vi "gu_message_box.vi"(7 "Title":T3, 8 "error in":errorcluster, 9 "Icon":T1, 10 "Choice":T2, 11 "Message":T3) -> (0 "error out":errorcluster, 3 "Button":T4=enum."Cancel")   [LabVIEW 2020, in "G-Unicode.lvlib"]
uses:
  G-Unicode.lvlib
  Dialog & User Interface/Message Box/Message Box Dialog Button.ctl
  Types/Encoded UTF-8 String.ctl
  Dialog & User Interface/Message Box/Message Box Dialog Type.ctl
  Dialog & User Interface/Message Box/Message Box Icon Type.ctl
  <vilib>/Utility/file.llb/Application Directory.vi
  <vilib>/Utility/error.llb/Error Cluster From Error Code.vi
  lib/g_unicode_32.dll
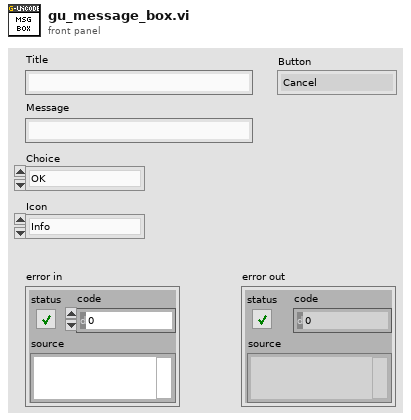
[diagram p1: front panel]
types:
  T1 = typedef "G-Unicode.lvlib/Message Box Icon Type.ctl" = enum16{"Info", "Warning", "Error", "Question"}
  T2 = typedef "G-Unicode.lvlib/Message Box Dialog Type.ctl" = enum32{"OK", "OK/Cancel", "Yes/No", "Yes/No/Cancel", "Retry/Cancel", "Abort/Retry/Ignore"}
  T3 = typedef "G-Unicode.lvlib/Encoded UTF-8 String.ctl" = string
  T4 = typedef "G-Unicode.lvlib/Message Box Dialog Button.ctl" = enum32{"OK", "Yes", "No", "Abort", "Retry", "Ignore", "Cancel"}
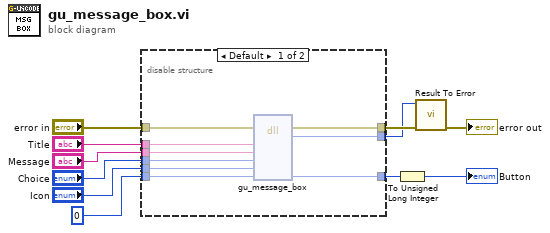
[diagram p0: block diagram]
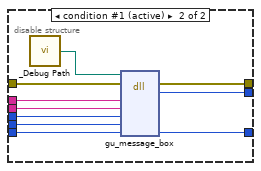
[diagram p2: hidden frame]
diagram:
  n1 = disable-structure shown="Default" {
    disable-tunnel: [w20 w30] -> w11
    disable-tunnel: [w14 w22] -> w10
    disable-tunnel: "Title" -> [w19 w29]
    disable-tunnel: "error in" -> [w18 w28]
    disable-tunnel: "Message" -> [w17 w27]
    disable-tunnel: "Choice" -> [w16 w26]
    disable-tunnel: "Icon" -> [w15 w25]
    disable-tunnel: [w13 w21] -> w2
    disable-tunnel: 0 ("user_selection") -> [w12 w23]
    frame condition #0 {
      n2 = dll-call lib="C:/github/dataflowg/g-unicode/src/LabVIEW/G-Unicode/lib/g_unicode_*.*" fn="gu_message_box"(error in=w18, "title"=w19, "message"=w17, "choice"=w16, "icon"=w15, "user_selection"=w12) -> (error out=w20:errorcluster, "result"=w13:i32, "user_selection"=w14:i32)  [unwired: 6 in, 1 out]
    }
    frame condition #1 (active) {
      n3 = call "_Debug Path.vi"() -> ("Debug Path"=w24:path)
      n4 = dll-call lib="?" fn="gu_message_box"(path in=w24, error in=w28, "title"=w29, "message"=w27, "choice"=w26, "icon"=w25, "user_selection"=w23) -> (error out=w30:errorcluster, "result"=w21:i32, "user_selection"=w22:i32)  [unwired: 5 in, 1 out]
    }
  }
  n5 = To Unsigned Long Integer(number=w10) -> (unsigned 32bit integer=→"Button":u32)
  n6 = call "Result To Error.vi"("error in (no error)"=w11, "Result Code"=w2) -> ("error out"=→"error out":errorcluster)  [unwired: 9 in]
